vi "id.From JSON Tree.vi"(8 "error in (no error)":errorcluster, 10 "JSON Value in":variant, 11 "id in":refnum<class "id.lvclass">) -> (0 "error out":errorcluster, 3 "id out":refnum<class "id.lvclass">)   [LabVIEW 2020, in "JSON-RPC Lib.lvlib" / "id.lvclass"]
uses:
  id.lvclass
  id.lvclass/id.ctl
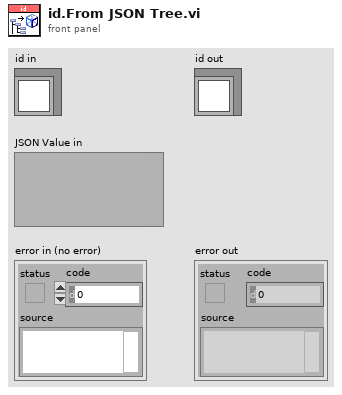
[diagram p1: front panel]
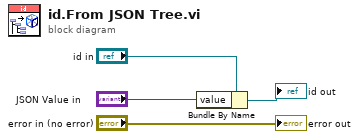
[diagram p0: block diagram]
diagram:
  n1 = Bundle By Name(cluster="id in", "value"="JSON Value in") -> (→"id out":refnum<class "id.lvclass">)
  "error out" <- "error in (no error)"
